vi "FlatToRichrfcontrol_SetTriggerWaitRequest.vi"(5 "OutputClusterType":T1, 11 "InputCluster":T2) -> (3 "OutputCluster":T1)   [LabVIEW 2024, in "FlexSDR_gRPC_client.lvlib"]
uses:
  rfcontrol_SetTriggerWaitRequest_Flat.ctl
  rfcontrol_SetTriggerWaitRequest.ctl
  FlexSDR_gRPC_client.lvlib
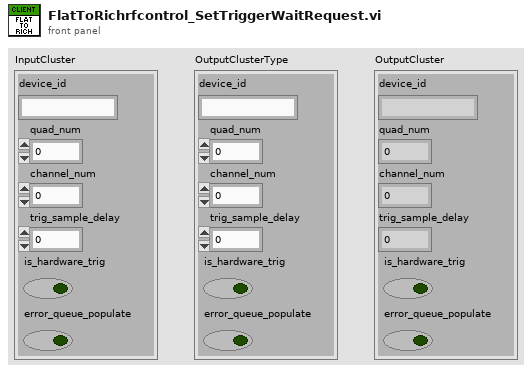
[diagram p1: front panel]
types:
  T1 = typedef "FlexSDR_gRPC_client.lvlib/rfcontrol_SetTriggerWaitRequest.ctl" = cluster{"device_id":string, "quad_num":i32, "channel_num":i32, "trig_sample_delay":i32, "is_hardware_trig":bool, "error_queue_populate":bool}
  T2 = typedef "FlexSDR_gRPC_client.lvlib/rfcontrol_SetTriggerWaitRequest_Flat.ctl" = cluster{"device_id":string, "quad_num":i32, "channel_num":i32, "trig_sample_delay":i32, "is_hardware_trig":bool, "error_queue_populate":bool}
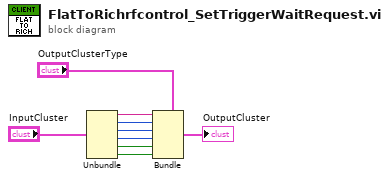
[diagram p0: block diagram]
diagram:
  n1 = Unbundle "Unbundle"("InputCluster") -> ("device_id"=w6:string, "quad_num"=w5:i32, "channel_num"=w4:i32, "trig_sample_delay"=w3:i32, "is_hardware_trig"=w2:bool, "error_queue_populate"=w1:bool)
  n2 = Bundle "Bundle"(cluster="OutputClusterType", "device_id"=w6, "quad_num"=w5, "channel_num"=w4, "trig_sample_delay"=w3, "is_hardware_trig"=w2, "error_queue_populate"=w1) -> (→"OutputCluster":T1)
